vi "flash.vi"() -> ()   [LabVIEW 2017]
panel:
  out "error out 3":errorcluster={"status"=TRUE, "code"=56, "source"="UDP Read in UDP.vi->flash.vi"}
  out "index 2":i32
  out "length":i32=256
  in  "FAST":bool=TRUE
  out "字符串":string
  out "error out 2":errorcluster
  in  "error in (no error)":errorcluster
  in  "Read (TRUE)":bool
  in  "IP address":string="192.168.10.20"
  in  "display":bool=TRUE
  out "index":i32
  out "data":string
  out "String":string
  out "size (in bytes)":i64=1443180
  out "In":u8=48 format="%x"
  in  "file path (use dialog)":path=path "G:/fpga_tdc/golden/golden.runs/impl_1/top_hdl.bin"
  out "error out":errorcluster={"status"=TRUE, "code"=56, "source"="UDP Read in UDP.vi->flash.vi"}
  in  "address":string="192.168.10.20"
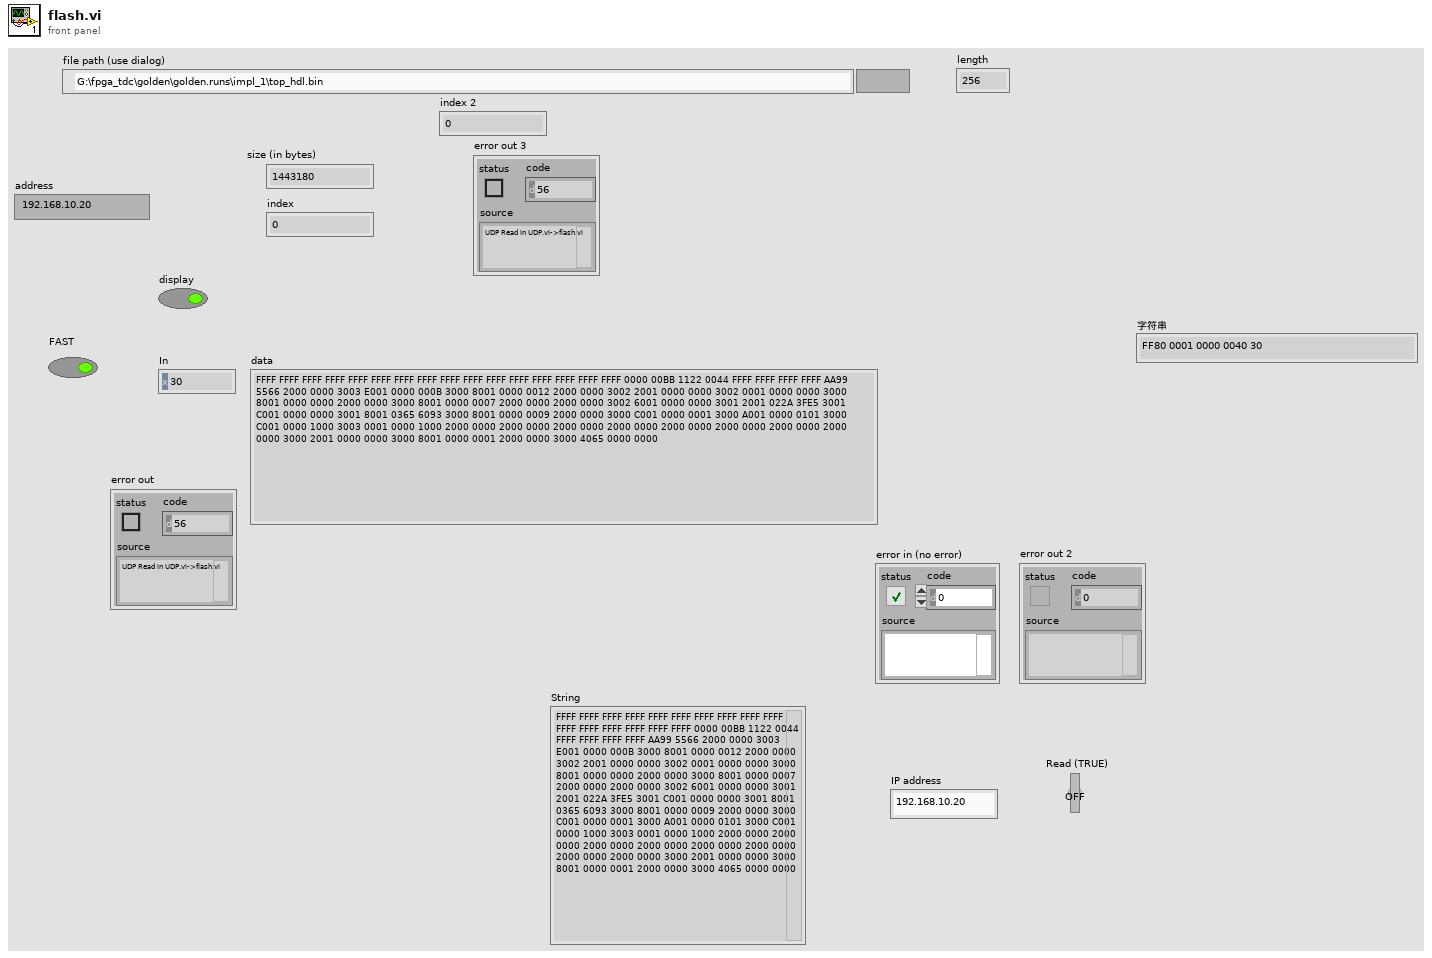
[diagram p1: front panel]
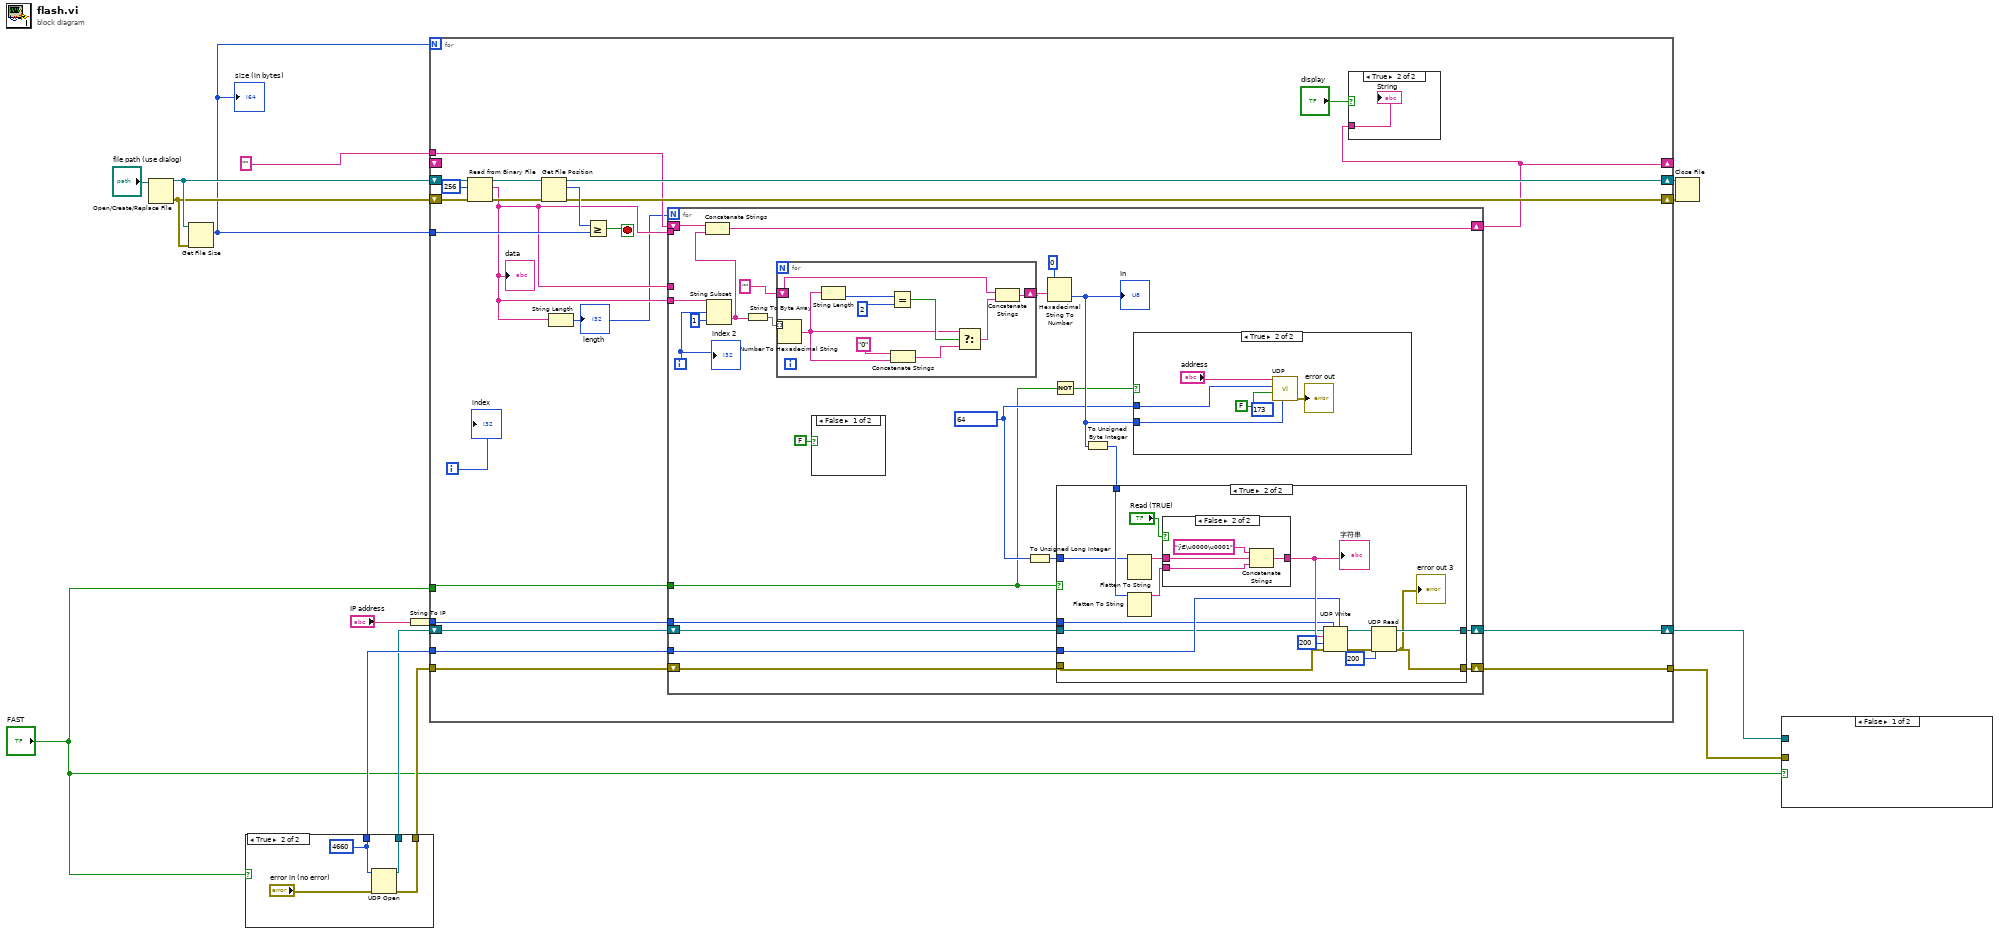
[diagram p0: block diagram]
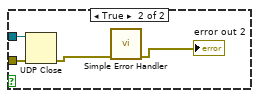
[diagram p2: hidden frame]
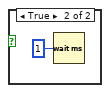
[diagram p4: hidden frame]
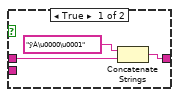
[diagram p6: hidden frame]
diagram:
  n1 = Open/Create/Replace File(file path (use dialog)="file path (use dialog)") -> (refnum out=w14:refnum<file>, error out=w13:errorcluster)  [unwired: 5 in, 1 out]
  n2 = Get File Size(file=w14, error in=w13) -> (size (in bytes)=w10:i64)  [unwired: 2 out]
  "size (in bytes)" <- w10
  n3 = case shown="True" "FAST" {
    tunnel: [_ w18] -> w9
    tunnel: [_ w17] -> w8
    tunnel: [_ w16] -> w7
    frame False {
    }
    frame True {
      w18 = u16 4660 ("UDP port")
      n4 = UDP Open(8:"error in (no error)", 11:w18) -> (port=w16:refnum<k16>, 0:w17:errorcluster)  [unwired: 3 in, 1 out]
    }
  }
  n5 = String To IP(1:"IP address") -> (0:w3:u32)
  n6 = for {
    N: w10 -> [_]
    tunnel: w10 -> [w36]
    shift-right: [w34] -> w12
    shift-left: w13 -> [w41]
    shift-right: [w33] -> w11
    shift-left: w14 -> [w42]
    shift-right: [w21] -> _
    shift-left: _ -> [_]
    tunnel: w9 -> [w30]
    tunnel: w8 -> [w29]
    tunnel: [w26] -> w5
    tunnel: w3 -> [w25]
    tunnel: "FAST" -> [w24]
    shift-right: [w27] -> w6
    shift-left: w7 -> [w28]
    tunnel: "" -> [w23]
    i -> [w32]
    stop <- w35 stop-if-true
    n7 = Read from Binary File(8:w41, 10:256 ("count (1)"), 11:w42) -> (0:w38:errorcluster, 2:w22:string, 3:w39:refnum<file>)  [unwired: 3 in, 1 out]
    "data" <- w22
    n8 = Get File Position(4:w38, 7:w39) -> (0:w34:errorcluster, 2:w37:i64, 3:w33:refnum<file>)
    n9 = String Length(string=w22) -> (length=w20:i32)
    "length" <- w20
    n10 = Greater Or Equal?(x=w37, y=w36) -> (x >= y?=w35:bool)
    n11 = for {
      N: w20 -> [_]
      tunnel: w30 -> [w61]
      tunnel: w25 -> [w56]
      tunnel: w24 -> [w50]
      tunnel: w22 -> [_]
      shift-right: [w57] -> w26
      shift-left: w29 -> [w60]
      shift-right: [w58] -> w27
      shift-left: w28 -> [w59]
      tunnel: w22 -> [w49]
      tunnel: w22 -> [_]
      shift-right: [w46] -> w21
      shift-left: w23 -> [w47]
      i -> [w43]
      w54 = u32 64 ("Address")
      n12 = String Subset(string=w49, offset (0)=w43, length (rest)=1 ("length (rest)")) -> (substring=w45:string)
      n13 = Concatenate Strings(w47, w45) -> (w46:string)
      n14 = String To Byte Array(string=w45) -> (unsigned byte array=w64:u8[])
      n15 = for {
        shift-right: [w105] -> w63
        shift-left: "" ("format string") -> [w102]
        tunnel: w64 -> [w106] mode=indexing
        n16 = Number To Hexadecimal String(2:w106) -> (0:w98:string)  [unwired: 1 in]
        n17 = String Length(string=w98) -> (length=w104:i32)
        n18 = Equal?(x=w104, y=2) -> (x = y?=w101:bool)
        n19 = Concatenate Strings("0" ("format string"), w98) -> (w100:string)
        n20 = Select(t=w98, s=w101, f=w100) -> (s? t:f=w97:string)
        n21 = Concatenate Strings(w102, w97) -> (w105:string)
      }
      n22 = case shown="False" FALSE {
        frame False {
        }
        frame True {
          n23 = Wait (ms)(milliseconds to wait=u32 1) -> ()  [unwired: 1 out]
        }
      }
      n24 = To Unsigned Long Integer(number=w54) -> (unsigned 32bit integer=w52:u32)
      n25 = Hexadecimal String To Number(string=w63, default (0uL)=u64 0 ("default (0 U32)")) -> (number=w55:u64)  [unwired: 1 in, 1 out]
      "In" <- w55
      n26 = Not(x=w50) -> (.not. x?=w51:bool)
      n27 = To Unsigned Byte Integer(number=w55) -> (unsigned 8bit integer=w53:u8)
      n28 = case shown="True" w50 {
        tunnel: w61 -> [_ w80]
        tunnel: w60 -> [w68 w79]
        tunnel: w59 -> [w67 w78]
        tunnel: [w67 w72] -> w58
        tunnel: [w68 w69] -> w57
        tunnel: w56 -> [_ w77]
        tunnel: w53 -> [_ w76]
        tunnel: w52 -> [_ w75]
        frame False {
        }
        frame True {
          n29 = Flatten To String(anything=w75) -> (data string=w83:string)  [unwired: 3 in, 2 out]
          n30 = Flatten To String(anything=w76) -> (data string=w82:string)  [unwired: 3 in, 2 out]
          n31 = case shown="False" "Read (TRUE)" {
            tunnel: [w86 w90] -> w84
            tunnel: w83 -> [w85 w89]
            tunnel: w82 -> [_ w88]
            frame True {
              n32 = Concatenate Strings("ÿÀ\u0000\u0001" ("initial string"), w85) -> (w86:string)
            }
            frame False {
              n33 = Concatenate Strings("ÿ€\u0000\u0001" ("initial string"), w89, w88) -> (w90:string)
            }
          }
          "字符串" <- w84
          n34 = UDP Write(address=w77, port or service name=w80, connection ID=w78, data in=w84, 8:w79, 9:200 ("timeout ms (25000)")) -> (error out=w71:errorcluster, 3:w73:refnum<k16>)
          n35 = UDP Read(connection ID=w73, timeout ms (25000)=200, 8:w71) -> (error out=w69:errorcluster, 3:w72:refnum<k16>)  [unwired: 4 out]
          "error out 3" <- w69
        }
      }
      n36 = case shown="True" w51 {
        tunnel: w55 -> [_ w93]
        tunnel: w54 -> [_ w92]
        frame False {
        }
        frame True {
          (unwired) u8 173 ("In")
          n37 = call "UDP.vi"("In"=w93, "Read (TRUE)"=FALSE, "Address"=w92, "IP address"="address") -> ("error out"=→"error out":errorcluster)  [unwired: 5 in, 1 out]
        }
      }
      "index 2" <- w43
    }
    n38 = case shown="True" "display" {
      tunnel: w21 -> [_ w107]
      frame False {
      }
      frame True {
        "String" <- w107
      }
    }
    "index" <- w32
  }
  n39 = Close File(refnum=w11, error in=w12) -> ()  [unwired: 2 out]
  n40 = case shown="False" "FAST" {
    tunnel: w6 -> [_ w109]
    tunnel: w5 -> [_ w108]
    frame False {
    }
    frame True {
      n41 = UDP Close(connection ID=w109, 8:w108) -> (error out=w111:errorcluster)  [unwired: 1 out]
      n42 = call <vilib>:"Simple Error Handler.vi"("error in (no error)"=w111) -> ("error out"=→"error out 2":errorcluster)  [unwired: 4 in, 4 out]
    }
  }
